vi "SystemVolume.Get.vi"(6 "Mode":i32(ring)=2 items=["Render", "Capture", "All"], 8 "error in (no error)":errorcluster, 11 "FriendlyName (\"\": All)":string) -> (0 "error out":errorcluster, 2 "FriendlyNames":string[](array[string]), 3 "Volumes":i32[](array[numeric]))   [LabVIEW 2014]
uses:
  C:/Program Files (x86)/National Instruments/LabVIEW 2014/user.lib/dge-library/LabVIEW/System/SystemVolume/NAudio.dll
  NAudio.dll
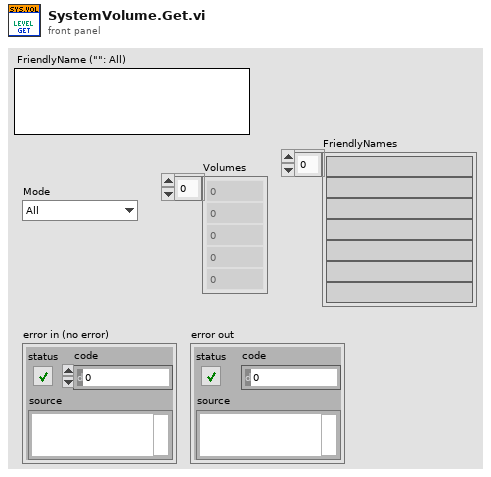
[diagram p1: front panel]
types:
  T1 = cluster{"AudioClient":refnum<k24>, "AudioEndpointVolume":refnum<k24>, "AudioMeterInformation":refnum<k24>, "AudioSessionManager":refnum<k24>, "DataFlow":i32, "DeviceFriendlyName":string, "FriendlyName":string, "IconPath":string, "ID":string}[]
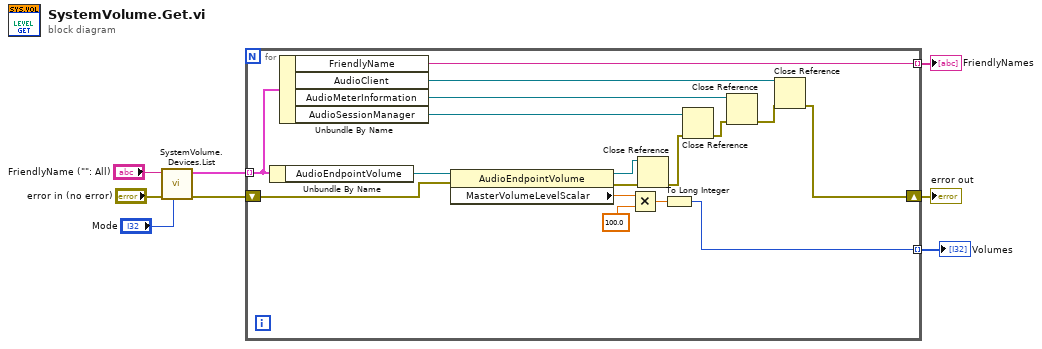
[diagram p0: block diagram]
diagram:
  n1 = call <userlib>:"SystemVolume.Devices.List.vi"("dataFlow"="Mode", "error in (no error)"="error in (no error)", "FriendlyName (\"\": All)"="FriendlyName (\"\": All)") -> ("error out"=w7:errorcluster, "Info"=w8:T1)  [unwired: 7 in]
  n2 = for {
    tunnel: w8 -> [w20] mode=indexing
    shift-right: [w13] -> w6
    shift-left: w7 -> [w12]
    tunnel: [w9] -> w4 mode=indexing
    tunnel: [w10] -> w3 mode=indexing
    n3 = Unbundle By Name(w20) -> ("AudioEndpointVolume"=w21:refnum<k24>)
    n4 = Unbundle By Name(w20) -> ("FriendlyName"=w10:string, "AudioClient"=w19:refnum<k24>, "AudioMeterInformation"=w18:refnum<k24>, "AudioSessionManager"=w16:refnum<k24>)
    n5 = property class="AudioEndpointVolume"(reference=w21, error in=w12) -> (reference out=w25:refnum<k24>, error out=w24:errorcluster, "MasterVolumeLevelScalar"=w22:sgl)
    n6 = Multiply(x=w22, y=sgl 100.0) -> (x*y=w11:sgl)
    n7 = Close Reference(reference=w25, error in (no error)=w24) -> (error out=w14:errorcluster)
    n8 = To Long Integer(number=w11) -> (32bit integer=w9:i32)
    n9 = Close Reference(reference=w16, error in (no error)=w14) -> (error out=w15:errorcluster)
    n10 = Close Reference(reference=w18, error in (no error)=w15) -> (error out=w17:errorcluster)
    n11 = Close Reference(reference=w19, error in (no error)=w17) -> (error out=w13:errorcluster)
  }
  "error out" <- w6
  "Volumes" <- w4
  "FriendlyNames" <- w3
